vi "Lab 6 I.vi"() -> ()   [LabVIEW 2021]
panel:
  out "?":bool
  in  "?":bool
  in  "Password:":string
  in  "Username:":string
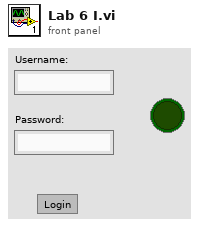
[diagram p1: front panel]
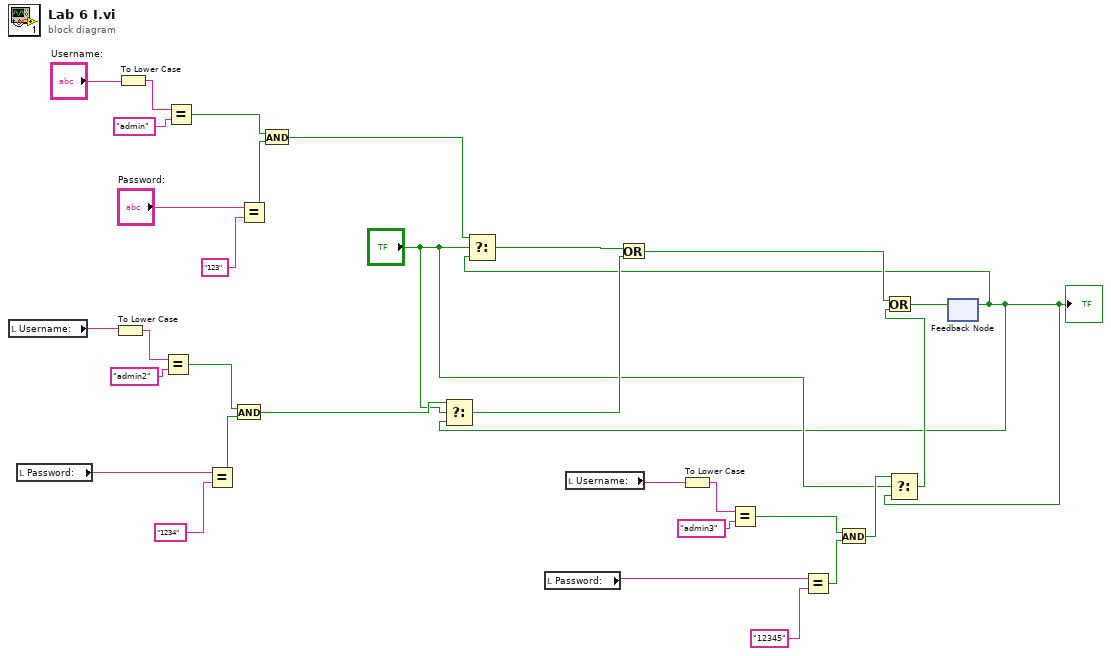
[diagram p0: block diagram]
diagram:
  n1 = local read "Username:"() -> (w22:string)
  n2 = local read "Password:"() -> (w20:string)
  n3 = To Lower Case(string=w22) -> (all lower case string=w24:string)
  n4 = To Lower Case(string="Username:") -> (all lower case string=w30:string)
  n5 = Equal?(x=w24, y="admin2") -> (x = y?=w19:bool)
  n6 = Equal?(x=w30, y="admin") -> (x = y?=w26:bool)
  n7 = Equal?(x=w20, y="1234") -> (x = y?=w18:bool)
  n8 = And(x=w19, y=w18) -> (x .and. y?=w15:bool)
  n9 = Equal?(x="Password:", y="123") -> (x = y?=w25:bool)
  n10 = And(x=w26, y=w25) -> (x .and. y?=w17:bool)
  n11 = local read "Password:"() -> (w10:string)
  n12 = local read "Username:"() -> (w9:string)
  n13 = To Lower Case(string=w9) -> (all lower case string=w13:string)
  n14 = Equal?(x=w13, y="admin3") -> (x = y?=w7:bool)
  n15 = Equal?(x=w10, y="12345") -> (x = y?=w8:bool)
  n16 = And(x=w7, y=w8) -> (x .and. y?=w6:bool)
  n17 = feedback #1() -> (w1:bool)  [unwired: 1 in]
  "?" <- w1
  n18 = Select(t=w15, s="?", f=w1) -> (s? t:f=w14:bool)
  n19 = Select(t=w17, s="?", f=w1) -> (s? t:f=w16:bool)
  n20 = Or(x=w16, y=w14) -> (x .or. y?=w4:bool)
  n21 = Select(t=w6, s="?", f=w1) -> (s? t:f=w3:bool)
  n22 = Or(x=w4, y=w3) -> (x .or. y?=w2:bool)
  n23 = feedback-in #1(w2) -> ()
